vi "Popcorn.vi"(11 "Boolean":bool) -> (3 "Boolean 2":bool)   [LabVIEW 2020]
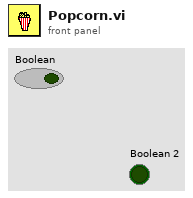
[diagram p1: front panel]
types:
  T1 = typedef "Sound Output Task ID.ctl" = u32
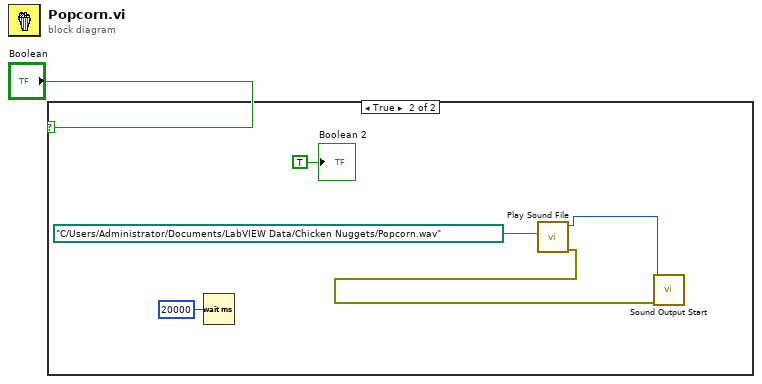
[diagram p0: block diagram]
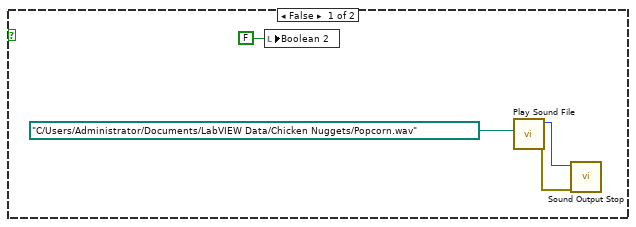
[diagram p2: hidden frame]
diagram:
  n1 = case shown="True" "Boolean" {
    frame False {
      n2 = local write "Boolean 2"(FALSE ("Boolean 2")) -> ()
      n3 = call <vilib>:"Play Sound File.vi"("path"=path "C:/Users/Administrator/Documents/LabVIEW Data/Chicken Nuggets/Popcorn.wav") -> ("error out"=w2:errorcluster, "task ID"=w3:T1)  [unwired: 9 in]
      n4 = call <vilib>:"Sound Output Stop.vi"("error in (no error)"=w2, "task ID"=w3) -> ()  [unwired: 8 in, 2 out]
    }
    frame True {
      n5 = Wait (ms)(milliseconds to wait=u32 20000) -> ()  [unwired: 1 out]
      n6 = call <vilib>:"Play Sound File.vi"("path"=path "C:/Users/Administrator/Documents/LabVIEW Data/Chicken Nuggets/Popcorn.wav") -> ("error out"=w8:errorcluster, "task ID"=w7:T1)  [unwired: 9 in]
      n7 = call <vilib>:"Sound Output Start.vi"("error in (no error)"=w8, "task ID"=w7) -> ()  [unwired: 8 in, 2 out]
      "Boolean 2" <- TRUE ("Boolean 2")
    }
  }
